vi "getTelemetryHardpointData.vi"(11 "Publisher in":refnum<class "Publisher.lvclass">) -> (2 "TelemetryHardpointData":T1, 3 "Publisher out":refnum<class "Publisher.lvclass">)   [LabVIEW 2016, in "Publisher.lvclass"]
uses:
  Publisher.lvclass
  DataTypes/Topics/TelemetryHardpointData.ctl
  DataTypes/Topics/Parts/Timestamp.ctl
  Publisher.lvclass/Publisher.ctl
  DataTypes/Topics/M1M3SupportTopics.lvlib
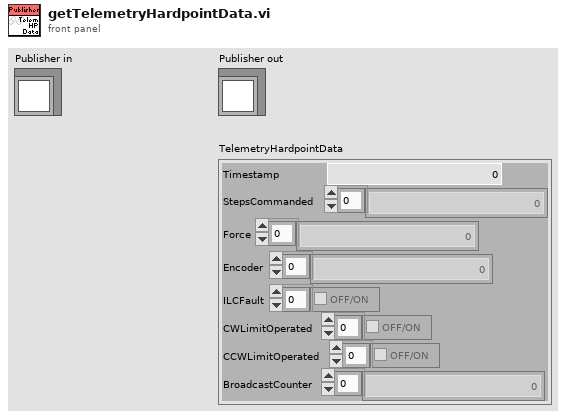
[diagram p1: front panel]
types:
  T1 = typedef "M1M3SupportTopics.lvlib/TelemetryHardpointData.ctl" = cluster{"Timestamp":T2, "StepsCommanded":i16[], "Force":sgl[], "Encoder":i32[], "ILCFault":bool[], "CWLimitOperated":bool[], "CCWLimitOperated":bool[], "BroadcastCounter":u8[]}
  T2 = typedef "M1M3SupportTopics.lvlib/Timestamp.ctl" = dbl
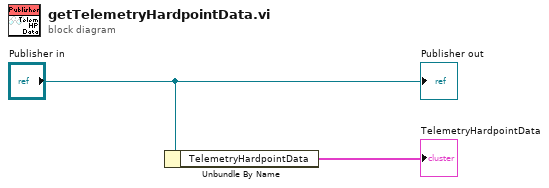
[diagram p0: block diagram]
diagram:
  n1 = Unbundle By Name("Publisher in") -> ("TelemetryHardpointData"=→"TelemetryHardpointData":T1)
  "Publisher out" <- "Publisher in"
